vi "MTS_ReadMSW.vi"(8 "error in (no error)":errorcluster, 11 "Workspace Path":path) -> (0 "error out":errorcluster, 1 "Created":string, 2 "Comment":string, 3 "Files in Workspace":T1(array[cluster]))   [LabVIEW 2011]
uses:
  <vilib>/Utility/config.llb/NI_LVConfig.lvlib
  <vilib>/Utility/config.llb/Read Key (String).vi
  <vilib>/Utility/config.llb/Read Key (I32).vi
  <vilib>/Utility/config.llb/Read Key (Double).vi
  <vilib>/Utility/config.llb/Read Key (Path).vi
  <vilib>/Utility/config.llb/Read Key (U32).vi
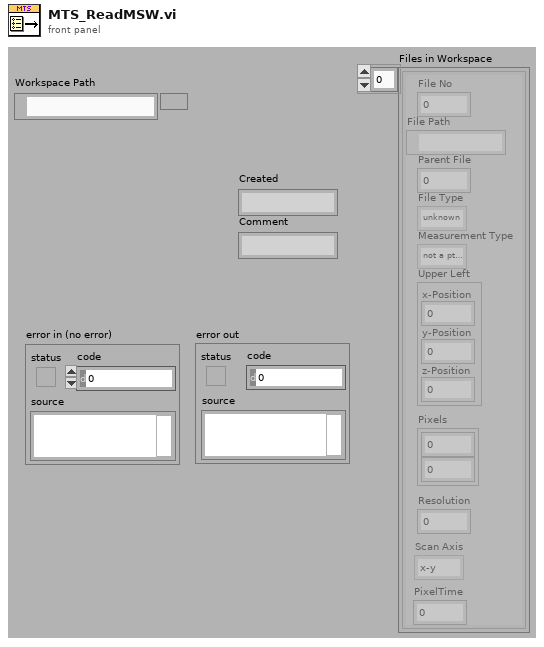
[diagram p1: front panel]
types:
  T1 = cluster{"File No":i32, "File Path":path, "Parent File":i32, "File Type":enum16{"unknown", "pt3 File", "png Image", "bmp Image"}, "Measurement Type":enum16{"not a pt3 File", "Image File", "Point Measurement", "Auto Point", "Line Scan", "Grid Scan"}, "Upper Left":cluster{"x-Position":dbl, "y-Position":dbl, "z-Position":dbl}, "Pixels":i32[], "Resolution":dbl, "Scan Axis":enum32{"x-y", "x-z", "y-z"}, "PixelTime":dbl}[]
  T2 = cluster{"File No":i32, "File Path":path, "Parent File":i32, "File Type":enum16{"unknown", "pt3 File", "png Image", "bmp Image"}, "Measurement Type":enum16{"not a pt3 File", "Image File", "Point Measurement", "Auto Point", "Line Scan", "Grid Scan"}, "Upper Left":cluster{"x-Position":dbl, "y-Position":dbl, "z-Position":dbl}, "Pixels":u16[], "Scan Axis":enum32{"x-y", "x-z", "y-z"}, "Resolution":dbl, dbl}
  T3 = typedef "NI_LVConfig.lvlib/Config Data RefNum.ctl" = refnum<k1>
  T4 = cluster{"File No":i32, "File Path":path, "Parent File":i32, "File Type":enum16{"unknown", "pt3 File", "png Image", "bmp Image"}, "Measurement Type":enum16{"not a pt3 File", "Image File", "Point Measurement", "Auto Point", "Line Scan", "Grid Scan"}, "Upper Left":cluster{"x-Position":dbl, "y-Position":dbl, "z-Position":dbl}, "Pixels":u16[], "Scan Axis":enum32{"x-y", "x-z", "y-z"}, "Resolution":dbl, dbl}[]
  T5 = enum16{"not a pt3 File", "Image File", "Point Measurement", "Auto Point", "Line Scan", "Grid Scan"}
  T6 = enum16{"unknown", "pt3 File", "png Image", "bmp Image"}
  T7 = cluster{i32, "value":path, "value":i32, "File Type":enum16{"unknown", "pt3 File", "png Image", "bmp Image"}, "Measurement Type":enum16{"not a pt3 File", "Image File", "Point Measurement", "Auto Point", "Line Scan", "Grid Scan"}, cluster{"value":dbl, "value":dbl, "value":dbl}, i32[], "value":dbl, "value":u32, "value":dbl}
  T8 = cluster{"File No":i32, "value":path, "value":i32, "File Type":enum16{"unknown", "pt3 File", "png Image", "bmp Image"}, "Measurement Type":enum16{"not a pt3 File", "Image File", "Point Measurement", "Auto Point", "Line Scan", "Grid Scan"}, "Upper Left":cluster{"value":dbl, "value":dbl, "value":dbl}, "Pixels":i32[], "value":dbl, "Resolution":dbl, "value":dbl}[]
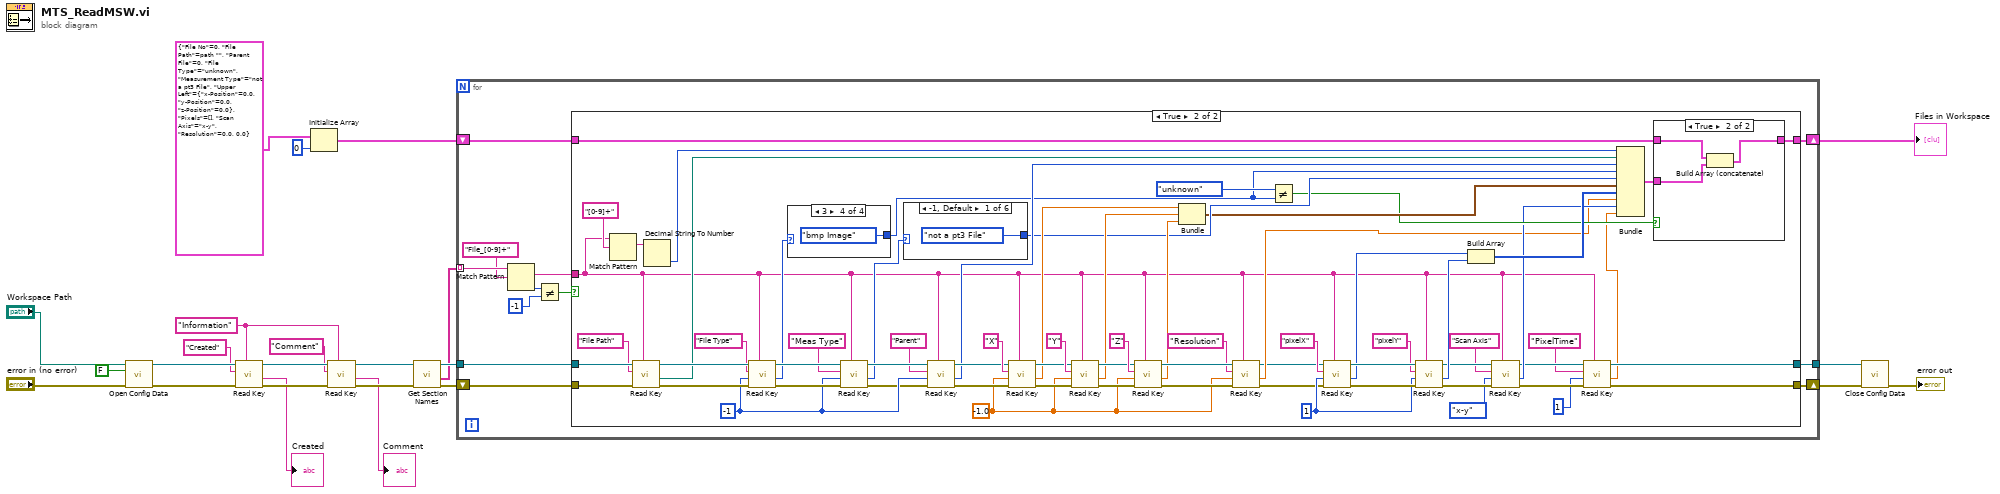
[diagram p0: block diagram]
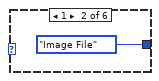
[diagram p4: hidden frame]
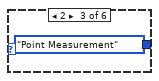
[diagram p5: hidden frame]
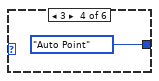
[diagram p6: hidden frame]
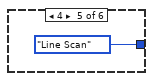
[diagram p7: hidden frame]
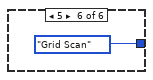
[diagram p8: hidden frame]
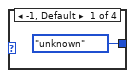
[diagram p9: hidden frame]
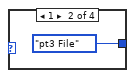
[diagram p10: hidden frame]
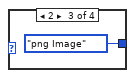
[diagram p11: hidden frame]
diagram:
  w16 = "Information" ("section")
  n1 = call <vilib>:"Open Config Data.vi"("error in (no error)"="error in (no error)", "create file if necessary (T)"=FALSE, "configuration file path"="Workspace Path") -> ("error out"=w21:errorcluster, "refnum"=w20:T3)  [unwired: 6 in, 1 out]
  n2 = call-poly <vilib>:"Read Key.vi"("section"=w16, "error in (no error)"=w21, "key"="Created", "refnum"=w20) -> ("error out"=w18:errorcluster, "value"=→"Created":string, "refnum out"=w17:T3)  [unwired: 4 in, 1 out]
  n3 = Initialize Array(T2 {"File No"=0, "File Path"=path "", "Parent File"=0, "File Type"=enum."unknown", "Measurement Type"=enum."not a pt3 File", "Upper Left"={"x-Position"=0.0, "y-Position"=0.0, "z-Position"=0.0}, "Pixels"=[], "Scan Axis"=enum."x-y", "Resolution"=0.0, 0.0} ("Cluster"), 0 ("dimension size")) -> (w4:T4)
  n4 = call-poly <vilib>:"Read Key.vi"("section"=w16, "error in (no error)"=w18, "key"="Comment", "refnum"=w17) -> ("error out"=w14:errorcluster, "value"=→"Comment":string, "refnum out"=w13:T3)  [unwired: 4 in, 1 out]
  n5 = call <vilib>:"Get Section Names.vi"("error in (no error)"=w14, "refnum"=w13) -> ("error out"=w12:errorcluster, "section names"=w10:string[], "refnum out"=w11:T3)  [unwired: 7 in]
  n6 = for {
    shift-right: [w28] -> w9
    shift-left: w12 -> [w30]
    tunnel: w11 -> [w29]
    tunnel: w10 -> [w36] mode=indexing
    tunnel: [w27] -> w8
    shift-right: [w25] -> w1
    shift-left: w4 -> [w26]
    n7 = Match Pattern(string=w36, regular expression="File_[0-9]+") -> (match substring=w31:string, offset past match=w34:i32)  [unwired: 1 in, 2 out]
    n8 = Not Equal?(x=w34, y=-1) -> (x != y?=w32:bool)
    n9 = case shown="True" w32 {
      tunnel: w31 -> [_ w42]
      tunnel: w30 -> [w39 w107]
      tunnel: w29 -> [w38 w106]
      tunnel: [w39 w46] -> w28
      tunnel: [w38 w44] -> w27
      tunnel: w26 -> [w37 w58]
      tunnel: [w37 w56] -> w25
      frame False {
      }
      frame True {
        w75 = 1 ("default value")
        w76 = -1.0 ("default value")
        w97 = -1 ("default value")
        n10 = Match Pattern(string=w42, regular expression="[0-9]+") -> (match substring=w98:string)  [unwired: 1 in, 3 out]
        n11 = call-poly <vilib>:"Read Key.vi"("section"=w42, "error in (no error)"=w107, "key"="File Path", "refnum"=w106) -> ("error out"=w104:errorcluster, "value"=w65:path, "refnum out"=w103:T3)  [unwired: 4 in, 1 out]
        n12 = Decimal String To Number(string=w98) -> (number=w66:i32)  [unwired: 2 in, 1 out]
        n13 = call-poly <vilib>:"Read Key.vi"("section"=w42, "error in (no error)"=w104, "default value"=w97, "key"="File Type", "refnum"=w103) -> ("error out"=w101:errorcluster, "value"=w69:i32, "refnum out"=w100:T3)  [unwired: 3 in, 1 out]
        n14 = case shown="3" w69 {
          tunnel: [T6."unknown" ("File Type") T6."pt3 File" ("File Type") T6."png Image" ("File Type") T6."bmp Image" ("File Type")] -> w63
          frame -1, Default {
          }
          frame 1 {
          }
          frame 2 {
          }
          frame 3 {
          }
        }
        n15 = call-poly <vilib>:"Read Key.vi"("section"=w42, "error in (no error)"=w101, "default value"=w97, "key"="Meas Type", "refnum"=w100) -> ("error out"=w96:errorcluster, "value"=w68:i32, "refnum out"=w95:T3)  [unwired: 3 in, 1 out]
        n16 = case shown="-1, Default" w68 {
          tunnel: [T5."not a pt3 File" ("Measurement Type") T5."Image File" ("Measurement Type") T5."Point Measurement" ("Measurement Type") T5."Auto Point" ("Measurement Type") T5."Line Scan" ("Measurement Type") T5."Grid Scan" ("Measurement Type")] -> w62
          frame -1, Default {
          }
          frame 1 {
          }
          frame 2 {
          }
          frame 3 {
          }
          frame 4 {
          }
          frame 5 {
          }
        }
        n17 = call-poly <vilib>:"Read Key.vi"("section"=w42, "error in (no error)"=w96, "default value"=w97, "key"="Parent", "refnum"=w95) -> ("error out"=w92:errorcluster, "value"=w64:i32, "refnum out"=w86:T3)  [unwired: 3 in, 1 out]
        n18 = call-poly <vilib>:"Read Key.vi"("section"=w42, "error in (no error)"=w92, "default value"=w76, "key"="X", "refnum"=w86) -> ("error out"=w91:errorcluster, "value"=w72:dbl, "refnum out"=w85:T3)  [unwired: 3 in, 1 out]
        n19 = call-poly <vilib>:"Read Key.vi"("section"=w42, "error in (no error)"=w91, "default value"=w76, "key"="Y", "refnum"=w85) -> ("error out"=w90:errorcluster, "value"=w71:dbl, "refnum out"=w84:T3)  [unwired: 3 in, 1 out]
        n20 = call-poly <vilib>:"Read Key.vi"("section"=w42, "error in (no error)"=w90, "default value"=w76, "key"="Z", "refnum"=w84) -> ("error out"=w83:errorcluster, "value"=w70:dbl, "refnum out"=w82:T3)  [unwired: 3 in, 1 out]
        n21 = Bundle("value"=w72, "value"=w71, "value"=w70) -> (w61:cluster{"value":dbl, "value":dbl, "value":dbl})  [unwired: 1 in]
        n22 = call-poly <vilib>:"Read Key.vi"("section"=w42, "error in (no error)"=w83, "default value"=w76, "key"="Resolution", "refnum"=w82) -> ("error out"=w49:errorcluster, "value"=w50:dbl, "refnum out"=w48:T3)  [unwired: 3 in, 1 out]
        n23 = Not Equal?(x=enum16{"unknown", "pt3 File", "png Image"}."unknown" ("File Type"), y=w63) -> (x != y?=w59:bool)
        n24 = call-poly <vilib>:"Read Key.vi"("section"=w42, "error in (no error)"=w49, "default value"=w75, "key"="pixelX", "refnum"=w48) -> ("error out"=w80:errorcluster, "value"=w74:i32, "refnum out"=w79:T3)  [unwired: 3 in, 1 out]
        n25 = call-poly <vilib>:"Read Key.vi"("section"=w42, "error in (no error)"=w80, "default value"=w75, "key"="pixelY", "refnum"=w79) -> ("error out"=w55:errorcluster, "value"=w73:i32, "refnum out"=w54:T3)  [unwired: 3 in, 1 out]
        n26 = Build Array(w74, w73) -> (w60:i32[])
        n27 = call-poly <vilib>:"Read Key.vi"("section"=w42, "error in (no error)"=w55, "default value"=enum32{"x-y", "x-z", "y-z"}."x-y" ("Scan Axis"), "key"="Scan Axis", "refnum"=w54) -> ("error out"=w47:errorcluster, "value"=w51:u32, "refnum out"=w45:T3)  [unwired: 3 in, 1 out]
        n28 = call-poly <vilib>:"Read Key.vi"("section"=w42, "error in (no error)"=w47, "default value"=1, "key"="PixelTime", "refnum"=w45) -> ("error out"=w46:errorcluster, "value"=w40:dbl, "refnum out"=w44:T3)  [unwired: 3 in, 1 out]
        n29 = Bundle(w66, "value"=w65, "value"=w64, "File Type"=w63, "Measurement Type"=w62, w61, w60, "value"=w50, "value"=w51, "value"=w40) -> (w57:T7)  [unwired: 1 in]
        n30 = case shown="True" w59 {
          tunnel: w58 -> [w108 w111]
          tunnel: w57 -> [_ w110]
          tunnel: [w108 w109] -> w56
          frame False {
          }
          frame True {
            n31 = Build Array (concatenate)(w111, w110) -> (w109:T8)
          }
        }
      }
    }
  }
  "Files in Workspace" <- w1
  n32 = call <vilib>:"Close Config Data.vi"("error in (no error)"=w9, "refnum"=w8) -> ("error out"=→"error out":errorcluster)  [unwired: 8 in, 1 out]
